vi "UDP_Receive_NEW_20170828.vi"(9 "address":string="234.5.6.7", 11 "receiver port":u16=55555) -> (1 "output array":bool[][](array[boolean]), 2 "roadblock names":string[](array[string]), 3 "raw string data":string)   [LabVIEW 2016]
uses:
  <vilib>/Utility/tcp.llb/UDP Multicast Read-Only Open.vi
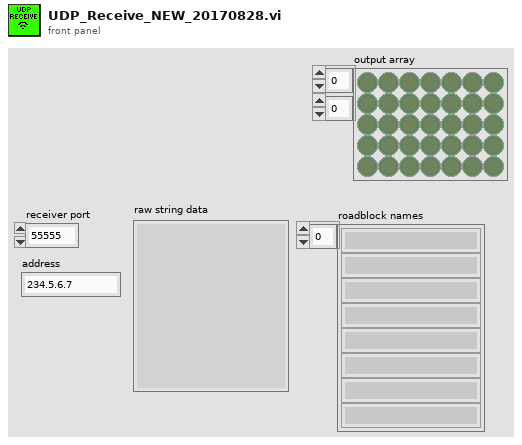
[diagram p1: front panel]
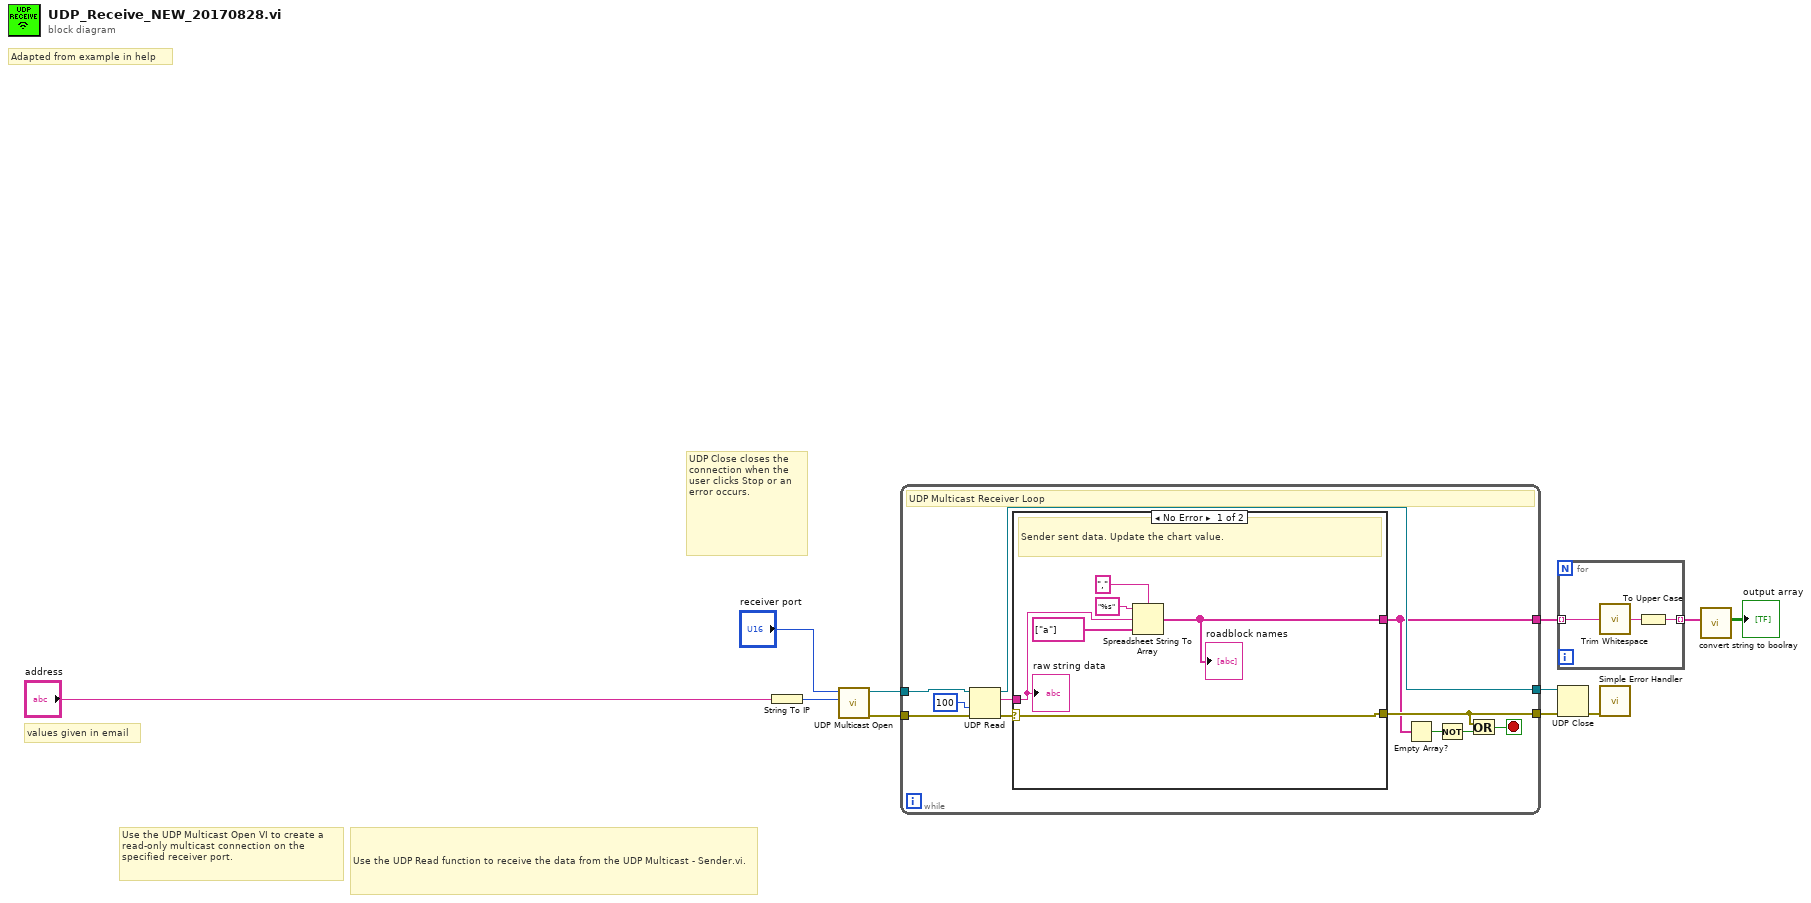
[diagram p0: block diagram]
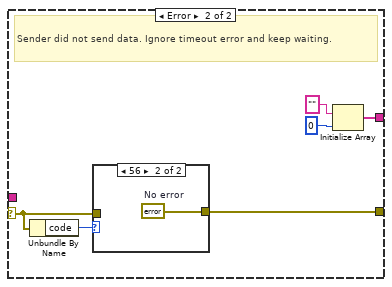
[diagram p2: hidden frame]
diagram:
  # "Adapted from example in help"
  # "UDP Close closes the connection when the user clicks Stop or an error occurs."
  # "Use the UDP Multicast Open VI to create a read-only multicast connection on the specified receiver port."
  # "values given in email"
  # "Use the UDP Read function to receive the data from the UDP Multicast - Sender.vi."
  n1 = String To IP(1:"address") -> (0:w4:u32)
  n2 = call-poly <vilib>:"UDP Multicast Open.vi"("multicast addr"=w4, "port"="receiver port") -> ("error out"=w7:errorcluster, "connection ID"=w6:refnum<k16>)  [unwired: 7 in, 1 out]
  n3 = while {
    tunnel: w6 -> [w22]
    tunnel: [w16] -> w11
    tunnel: w7 -> [w20]
    tunnel: [w15] -> w8
    tunnel: [w14] -> w2
    stop <- w21 stop-if-true
    # "UDP Multicast Receiver Loop"
    n4 = UDP Read(connection ID=w22, timeout ms (25000)=100, 8:w20) -> (data out=w18:string, error out=w17:errorcluster, 3:w16:refnum<k16>)  [unwired: 3 out]
    n5 = case shown="No Error" w17 {
      selector: w17 -> [w28 w33]
      tunnel: w18 -> [w25 _]
      tunnel: [w28 w32] -> w15
      tunnel: [w23 w30] -> w14
      frame No Error {
        # "Sender sent data. Update the chart value."
        n6 = Spreadsheet String To Array(delimiter (Tab)=",", format string="%s", spreadsheet string=w25, array type (2D Dbl)=string[] ["a"]) -> (array=w23:string[])
        "roadblock names" <- w23
        "raw string data" <- w25
      }
      frame Error {
        # "Sender did not send data. Ignore timeout error and keep waiting."
        n7 = Unbundle By Name(w33) -> ("code"=w34:i32)
        n8 = case shown="56" w34 {
          tunnel: w33 -> [w35 _]
          tunnel: [w35 w36] -> w32
          frame Default {
          }
          frame 56 {
            w36 = errorcluster {"status"=FALSE, "code"=0, "source"=""}  # No error
          }
        }
        n9 = Initialize Array("", 0 ("dimension size")) -> (w30:string[])
      }
    }
    n10 = Empty Array?(array=w14) -> (empty?=w13:bool)
    n11 = Not(x=w13) -> (.not. x?=w12:bool)
    n12 = Or(x=w15, y=w12) -> (x .or. y?=w21:bool)
  }
  n13 = for {
    tunnel: w2 -> [w39] mode=indexing
    tunnel: [w37] -> w1 mode=indexing
    n14 = call <vilib>:"Trim Whitespace.vi"("string"=w39) -> ("trimmed string"=w38:string)  [unwired: 1 in]
    n15 = To Upper Case(1:w38) -> (0:w37:string)
  }
  n16 = UDP Close(connection ID=w11, 8:w8) -> (error out=w9:errorcluster)  [unwired: 1 out]
  n17 = call <vilib>:"Simple Error Handler.vi"("error in (no error)"=w9) -> ()  [unwired: 1 in, 8 out]
  n18 = call "convert string to boolray.vi"("roadblock names"=w1) -> ("output array"=→"output array":bool[][])  [unwired: 10 in]
